vi "Actor Core.vi"(8 "error in":errorcluster, 11 "Nested in":refnum<class "Prooduct Actor.lvclass">) -> (0 "error out":errorcluster, 3 "Actor out":refnum<class "Actor.lvclass">)   [LabVIEW 2020, in "Prooduct Actor.lvlib" / "Prooduct Actor.lvclass"]
doc: "(<B>Filename</B>: Actor Framework.lvlib:Actor.lvclass:Actor Core.vi)\n\nReceives messages to the actor, reacts to them, and initiates any error handling that may shut the actor down.\n\nDescendant classes may override this VI to append parallel tasks for the actor to complete while it handles messages. Overrides use the Call Parent Method node."
uses:
  Prooduct Actor.lvclass
  C:/Program Files (x86)/National Instruments/LabVIEW 2020/vi.lib/ActorFramework/Actor/Actor.lvclass
  <vilib>/ActorFramework/Actor/Actor.lvclass
  Prooduct Actor.lvclass/Prooduct Actor.ctl
  <vilib>/ActorFramework/Actor/Actor.lvclass/Actor.ctl
  <vilib>/ActorFramework/Message Enqueuer/Message Enqueuer.lvclass/Message Enqueuer.ctl
  Prooduct Actor Messages/UpdateData Msg/UpdateData Msg.lvclass/UpdateData Msg.ctl
  Prooduct Actor Messages/ProductRequest Msg/ProductRequest Msg.lvclass/ProductRequest Msg.ctl
  Write VI Refnum.vi
  <vilib>/ActorFramework/Message Enqueuer/Init from Existing Queue.vi
  <vilib>/ActorFramework/Message Enqueuer/Enqueue.vi
  <vilib>/ActorFramework/Stop Msg/Stop Msg.lvclass
  C:/Program Files (x86)/National Instruments/LabVIEW 2020/vi.lib/ActorFramework/Message/Message.lvclass
  Prooduct Actor Messages/UpdateData Msg/UpdateData Msg.lvclass
  Prooduct Actor Messages/ProductRequest Msg/ProductRequest Msg.lvclass
  <vilib>/ActorFramework/Message Priority Queue/Priority Enqueue.vi
  <vilib>/ActorFramework/Message Enqueuer/Message Enqueuer.lvclass
panel:
  in  "Productos":i32(listbox)
  in  "Comprar":bool
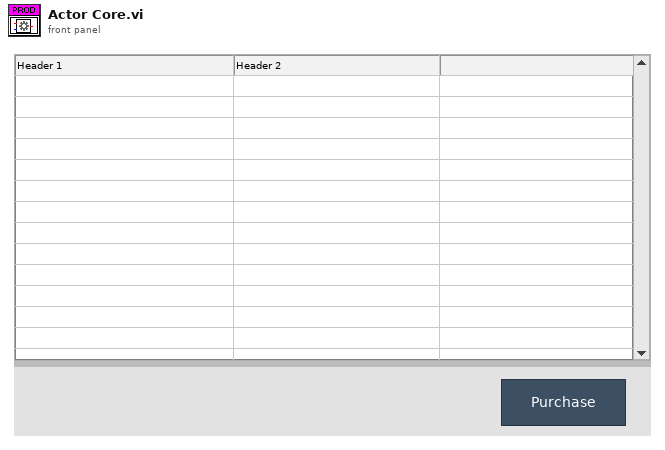
[diagram p1: front panel]
types:
  T1 = cluster{"Stop":refnum<user-event>, "ButtonLabel":refnum<user-event>, "Update List":refnum<user-event>}
  T2 = typedef "Currency Enum.ctl" = enum16{"USD", "MXN", "EUR"}
  T3 = typedef "Language Enum.ctl" = enum16{"English", "Español", "Français"}
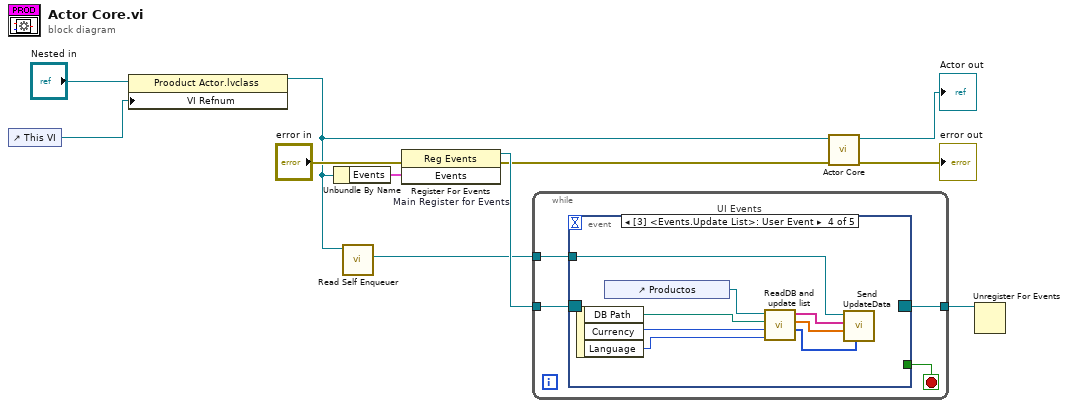
[diagram p0: block diagram]
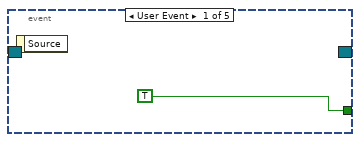
[diagram p2: hidden frame]
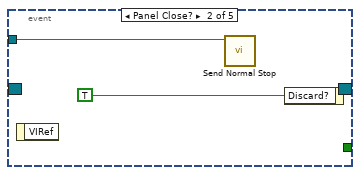
[diagram p3: hidden frame]
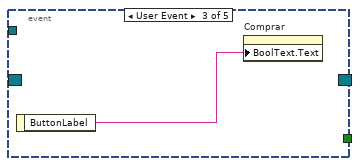
[diagram p4: hidden frame]
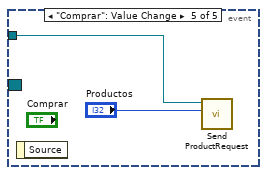
[diagram p5: hidden frame]
diagram:
  n1 = control-ref of="This VI"() -> (w1:refnum<vi>)
  n2 = property class="Prooduct Actor.lvclass"(reference="Nested in", "VI Refnum"=w1) -> (reference out=w2:refnum<class "Prooduct Actor.lvclass">)  [unwired: 1 in, 1 out]
  n3 = Unbundle By Name(w2) -> ("Events"=w8:T1)
  n4 = call <vilib>:"Read Self Enqueuer.vi"("Actor"=w2) -> ("Self Enqueuer"=w6:refnum<class "Message Enqueuer.lvclass">)  [unwired: 10 in]
  n5 = register-events "Main Register for Events"(error in="error in", w8) -> (reference out=w9:refnum<event-registration>, error out=w4:errorcluster)  [unwired: 1 in]
  n6 = while {
    tunnel: w9 -> [w15]
    tunnel: [w13] -> w7
    tunnel: w6 -> [w12]
    stop <- w14 stop-if-true
    n7 = event "UI Events" shown="[3] <Events.Update List>: User Event" {
      selector: w15 -> [_ _ _ _ _]
      dyn-events: [_ _ _ _ _] -> w13
      timeout: _ -> [_ _ _ _ _]
      tunnel: [TRUE _ _ _ _] -> w14
      tunnel: w12 -> [_ w17 _ w23 w29]
      event User Event {
        n8 = event-data() -> ()  [unwired: 1 in, 1 out]
      }
      event Panel Close? {
        n9 = event-data() -> ()  [unwired: 1 in, 1 out]
        n10 = call <vilib>:"Send Normal Stop.vi"("Message Enqueuer"=w17) -> ()  [unwired: 10 in, 1 out]
        n11 = event-data("Discard?"=TRUE) -> ()  [unwired: 1 in, 1 out]
      }
      event User Event {
        n12 = event-data() -> ("ButtonLabel"=w19:string)  [unwired: 1 in]
        n13 = property on="Comprar" class="Bool"("BoolText.Text"=w19) -> ()  [unwired: 2 in, 2 out]
      }
      event User Event {
        n14 = event-data() -> ("DB Path"=w26:path, "Currency"=w25:T2, "Language"=w24:T3)  [unwired: 1 in]
        n15 = control-ref of="Productos"() -> (w27:refnum<vi>)
        n16 = call "ReadDB and update list.vi"("Language"=w24, "Currency"=w25, "DB Path"=w26, "MCListbox Refnum"=w27) -> ("Quantity Array"=w20:i64[], "Prices Array"=w22:dbl[], "Names Array"=w21:string[])  [unwired: 5 in]
        n17 = call "Send UpdateData.vi"("Stock"=w20, "Prices"=w22, "Products"=w21, "Message Enqueuer"=w23) -> ()  [unwired: 6 in, 2 out]
      }
      event "Comprar": Value Change {
        n18 = event-data() -> ()  [unwired: 1 in, 1 out]
        n19 = call "Send ProductRequest.vi"("Product Index"="Productos", "Message Enqueuer"=w29) -> ()  [unwired: 8 in, 2 out]
      }
    }
  }
  n20 = call-parent "Actor Core.vi"("error in"=w4, "Actor in"=w2) -> ("error out"=→"error out":errorcluster, "Actor out"=→"Actor out":refnum<class "Actor.lvclass">)  [unwired: 8 in]
  n21 = Unregister For Events(event registration refnum=w7) -> ()  [unwired: 1 in, 1 out]
